vi "PUBLIC.constructor.vi"(0 "name":string, 2 "data in":string, 5 "error in (no error)":errorcluster) -> (14 "i ref out":refnum<vi>, 16 "data out":string, 19 "error out":errorcluster)   [LabVIEW 2014, in "NanotecSMCPD.lvlib"]
doc: "This is the constructor of a class.\n\nLicense Agreement for this software:\n\nCopyright (C)\nGesellschaft für Schwerionenforschung, GSI\nPlanckstr. 1\n64291 Darmstadt\nGermany\n\nContact: D.Beck@gsi.de \n\nThis program is free software; you can redistribute it and/or modify it under the terms of the \nGNU General Public License as published by the Free Software Foundation; either version 2 of \nthe license, or (at your option) any later version.\n\nThis program is distributed in the hope that it will be useful, but WITHOUT ANY WARRANTY; \nwithout even the implied warranty of MERCHANTABILITY or FITNESS FOR A PARTICULAR PURPOSE. See the GNU General License for more details (http://www.gnu.org).\n\nGesellschaft für Schwerionenforschung, GSI\nPlanckstr. 1, 64291 Darmstadt, Germany\nFor all questions and ideas contact: M.Richter@gsi.de, H.Brand@gsi.de or D.Beck@gsi.de.\nLast update: 16-JUN-2004"
uses:
  NanotecSMCPD.lvlib
  CSCore/CSApplicationBaseClasses/DeviceBase/DeviceBase.myEventNames.ctl
  CSCore/CSApplicationBaseClasses/MotorBase/MotorBase.myEventNames.ctl
  CSCore/CSSystem/CSSystemLib/CSSystemLib.lvlib
  CSCore/CSApplicationBaseClasses/DeviceBase/DeviceBase.lvlib
  CSCore/CSApplicationBaseClasses/MotorBase/MotorBase.lvlib
  CSCore/BaseProcess/BaseProcess.lvlib
  CSCore/CSObj/CSObj.lvlib
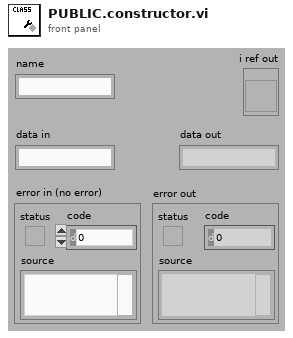
[diagram p1: front panel]
types:
  T1 = enum16{"SetAttribute", "GetAttribute", "CreateAttribute", "DestroyAttribute", "DestroyAllAtributes"}
  T2 = typedef "MotorBase.lvlib/MotorBase.myEventNames.ctl" = enum16{"lvmsg://SetDefaultAxisIndex", "lvmsg://GetDefaultAxisIndex", "lvmsg://GetNofAxes", "lvmsg://EmergencyOff", "lvmsg://SetOnOff", "lvmsg://GetOnOff", "lvmsg://SetStartVelocity", "lvmsg://GetStartVelocity", "lvmsg://SetStopVelocity", "lvmsg://GetStopVelocity", "lvmsg://SetAcceleration", "lvmsg://GetAcceleration", "lvmsg://SetRangeMin", "lvmsg://GetRangeMin", "lvmsg://SetRangeMax", "lvmsg://GetRangeMax", "lvmsg://GetStatus", "lvmsg://SetPosition", "lvmsg://GetPosition", "lvmsg://GetNames", "lvmsg://GetUnit", "lvmsg://ResetDefault", "lvmsg://MoveAbsolute", "lvmsg://MoveRelative", "lvmsg://Stop", "lvmsg://Halt", "lvmsg://FindReference", "lvmsg://SetAxisOnOff", "lvmsg://GetAxisOnOff", "lvmsg://SetAxisStartVelocity", "lvmsg://GetAxisStartVelocity", "lvmsg://SetAxisStopVelocity", "lvmsg://GetAxisStopVelocity", "lvmsg://SetAxisAcceleration", "lvmsg://GetAxisAcceleration", "lvmsg://SetAxisRangeMin", "lvmsg://GetAxisRangeMin", "lvmsg://SetAxisRangeMax", "lvmsg://GetAxisRangeMax", "lvmsg://GetAxisStatus", "lvmsg://SetAxisPosition", "lvmsg://GetAxisPosition", "lvmsg://GetAxisNames", "lvmsg://GetAxisUnit", "lvmsg://ResetAxis", "lvmsg://MoveAxisAbsolute", "lvmsg://MoveAxisRelative", "lvmsg://StopAxis", "lvmsg://HaltAxis", "lvmsg://FindAxisReference"}
  T3 = typedef "DeviceBase.lvlib/DeviceBase.myEventNames.ctl" = enum16{"lvmsg://Initialize", "lvmsg://Close", "lvmsg://Configure", "lvmsg://Reset", "lvmsg://IDQuery"}
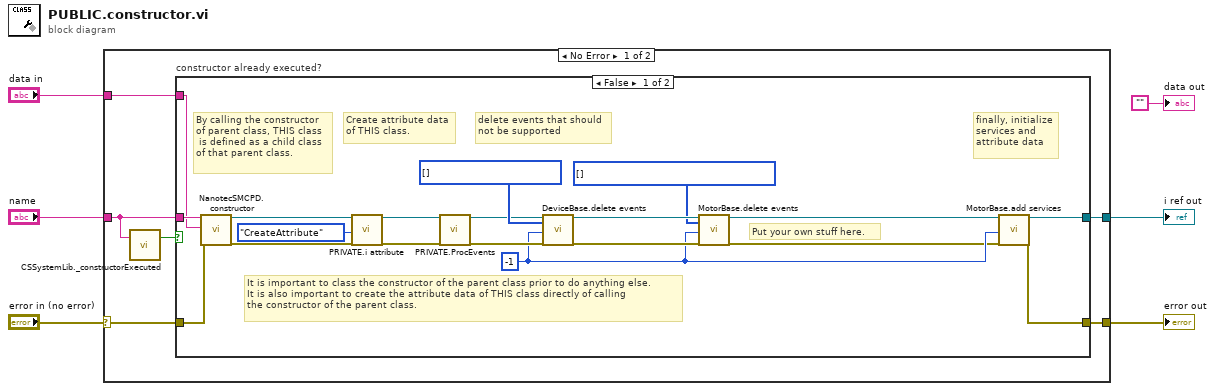
[diagram p0: block diagram]
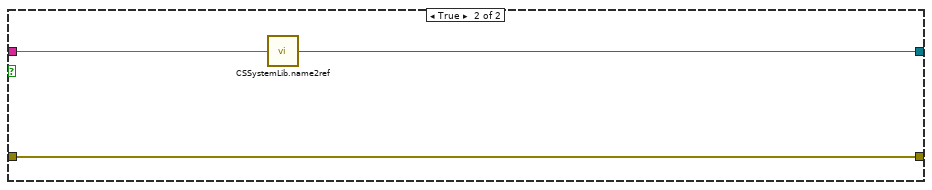
[diagram p2: hidden frame]
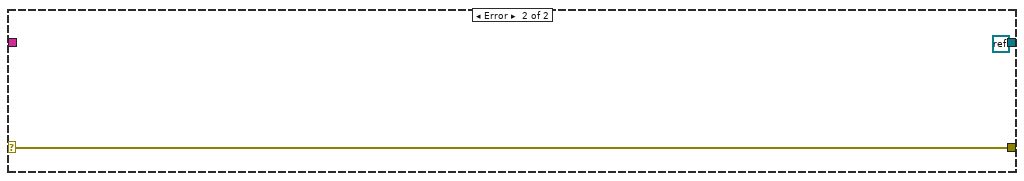
[diagram p3: hidden frame]
diagram:
  n1 = case shown="No Error" "error in (no error)" {
    selector: "error in (no error)" -> [w10 w35]
    tunnel: "name" -> [w9 _]
    tunnel: [w12 refnum<k0> refnum] -> w5
    tunnel: [w11 w35] -> w4
    tunnel: "data in" -> [w7 _]
    frame No Error {
      n2 = call "CSSystemLib._constructorExecuted.vi"("name"=w9) -> ("constructor executed?"=w8:bool)  [unwired: 18 in]
      n3 = case "constructor already executed?" shown="False" w8 {
        tunnel: w9 -> [w28 w34]
        tunnel: [w14 w33] -> w12
        tunnel: [w15 w32] -> w11
        tunnel: w10 -> [w25 w32]
        tunnel: w7 -> [w24 _]
        frame False {
          w13 = T2[] [] items=["lvmsg://SetDefaultAxisIndex", "lvmsg://GetDefaultAxisIndex", "lvmsg://GetNofAxes", "lvmsg://EmergencyOff", "lvmsg://SetOnOff", "lvmsg://GetOnOff", "lvmsg://SetStartVelocity", "lvmsg://GetStartVelocity", "lvmsg://SetStopVelocity", "lvmsg://GetStopVelocity", "lvmsg://SetAcceleration", "lvmsg://GetAcceleration", "lvmsg://SetRangeMin", "lvmsg://GetRangeMin", "lvmsg://SetRangeMax", "lvmsg://GetRangeMax", "lvmsg://GetStatus", "lvmsg://SetPosition", "lvmsg://GetPosition", "lvmsg://GetNames", "lvmsg://GetUnit", "lvmsg://ResetDefault", "lvmsg://MoveAbsolute", "lvmsg://MoveRelative", "lvmsg://Stop", "lvmsg://Halt", "lvmsg://FindReference", "lvmsg://SetAxisOnOff", "lvmsg://GetAxisOnOff", "lvmsg://SetAxisStartVelocity", "lvmsg://GetAxisStartVelocity", "lvmsg://SetAxisStopVelocity", "lvmsg://GetAxisStopVelocity", "lvmsg://SetAxisAcceleration", "lvmsg://GetAxisAcceleration", "lvmsg://SetAxisRangeMin", "lvmsg://GetAxisRangeMin", "lvmsg://SetAxisRangeMax", "lvmsg://GetAxisRangeMax", "lvmsg://GetAxisStatus", "lvmsg://SetAxisPosition", "lvmsg://GetAxisPosition", "lvmsg://GetAxisNames", "lvmsg://GetAxisUnit", "lvmsg://ResetAxis", "lvmsg://MoveAxisAbsolute", "lvmsg://MoveAxisRelative", "lvmsg://StopAxis", "lvmsg://HaltAxis", "lvmsg://FindAxisReference"] ("events")
          w23 = T3[] [] items=["lvmsg://Initialize", "lvmsg://Close", "lvmsg://Configure", "lvmsg://Reset", "lvmsg://IDQuery"] ("events")
          w17 = -1 ("ms timeout (10000)")
          # "finally, initialize\nservices and\nattribute data"
          # "delete events that should\nnot be supported"
          # "It is important to class the constructor of the parent class prior to do anything else.\nIt is also important to create the attribute data of THIS class directly of calling\nthe constructor of the parent class."
          # "Put your own stuff here."
          # "Create attribute data\nof THIS class."
          # "By calling the constructor\nof parent class, THIS class\n is defined as a child class\nof that parent class."
          n4 = call "NanotecSMCPD.constructor.vi"("name"=w28, "data in"=w24, "error in (no error)"=w25) -> ("i ref out"=w31:refnum<vi>, "error out"=w30:errorcluster)  [unwired: 14 in, 1 out]
          n5 = call "PRIVATE.i attribute.vi"("VI Refnum"=w31, "Action"=T1."CreateAttribute", "error in (no error)"=w30) -> ("VI Refnum out"=w27:refnum<vi>, "error out"=w26:errorcluster)  [unwired: 14 in, 1 out]
          n6 = call "PRIVATE.ProcEvents.vi"("i ref in"=w27, "error in (no error)"=w26) -> ("i ref out"=w22:refnum<vi>, "error out"=w21:errorcluster)  [unwired: 16 in]
          n7 = call "DeviceBase.delete events.vi"("i ref in"=w22, "events"=w23, "ms timeout (10000)"=w17, "error in (no error)"=w21) -> ("i ref out"=w20:refnum<vi>, "error out"=w18:errorcluster)  [unwired: 13 in, 1 out]
          n8 = call "MotorBase.delete events.vi"("i ref in"=w20, "events"=w13, "ms timeout (10000)"=w17, "error in (no error)"=w18) -> ("i ref out"=w19:refnum<vi>, "error out"=w16:errorcluster)  [unwired: 13 in, 1 out]
          n9 = call "MotorBase.add services.vi"("i ref in"=w19, "ms timeout (10000)"=w17, "error in (no error)"=w16) -> ("i ref out"=w14:refnum<vi>, "error out"=w15:errorcluster)  [unwired: 14 in, 1 out]
        }
        frame True {
          n10 = call "CSSystemLib.name2ref.vi"("name"=w34) -> ("obj refnum"=w33:refnum<vi>)
        }
      }
    }
    frame Error {
    }
  }
  "i ref out" <- w5
  "error out" <- w4
  "data out" <- ""
